vi "teleop_v2.vi"() -> ()   [LabVIEW 2012, in "MainProject.lvrbt"]
uses:
  MainProject.lvrbt
  <vilib>/NXT/Hardware/Plugins/Tetrix DC Motor/TetrixDCMotorAddress.ctl
  <vilib>/NXT/Dual Mode Library/Advanced/NXTFlag_Get_String.vi
  <vilib>/FTC/FTC Read Controller Packet.vi
  <vilib>/FTC/FTC Read Button States.vi
  <vilib>/NXT/NXTIO Xnodes/NXTIONodeSubVIs/TETRIX IO Move DC Motors.vi
  <vilib>/NXT/NXTIO Xnodes/NXTIONodeSubVIs/TETRIX IO Stop DC Motors.vi
  <vilib>/FTC/FTC Calculate Drive Power - Tank.vi
  <vilib>/NXT/Dual Mode Library/Advanced/NXTFlag_Assign_String.vi
  <vilib>/NXT/NXTIO Xnodes/NXTIONodeSubVIs/TETRIX IO Check Battery.vi
  <vilib>/NXT/NXTIO Xnodes/AddressXNode/NXTIOAddress.xnode
  <vilib>/NXT/Subs/LVHSConnector.ctl
  <vilib>/NXT/NXTIO Xnodes/NXTIOXNode/NXTIO.xnode
  <vilib>/NXT/LegoClasses/BrickReference/BrickReference.lvclass
panel:
  in  "Drive Power":i8=75 min=-100 max=100
  # "This VI was generated based on your configuration in the Remote Control Editor. You may modify the code as needed for your robot. To test this program for an FTC match, return to the Remote Control Editor, select the \"Run Program\" tab, and choose \"Teleop\"."
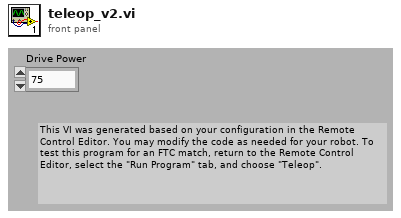
[diagram p1: front panel]
types:
  T1 = typedef "TetrixDCMotorAddress.ctl" = i16
  T2 = cluster{"TetrixDCMotor":T1, "TetrixDCMotor 2":T1}
  T3 = typedef "LVHSConnector.ctl" = refnum<class "BrickReference.lvclass">
  T4 = typedef "FTC ControllerState.ctl" = cluster{"Left X":i8, "Left Y":i8, "Right X":i8, "Right Y":i8, "Button Encoding 9-12":u8, "Button Encoding 1-8":u8, "POV":T5}
  T5 = typedef "FTC POVState.ctl" = i8
  T6 = typedef "FTC ButtonEventType.ctl" = enum16{"Pressed", "Released"}
  T7 = cluster{"Button ID":enum16{"None", "Button 1", "Button 2", "Button 3", "Button 4", "Button 5", "Button 6", "Button 7", "Button 8", "Button 9", "Button 10", "Button 11", "Button 12", "POV Up", "POV Up Right", "POV Right", "POV Down Right", "POV Down", "POV Down Left", "POV Left", "POV Up Left"}, "Event Type":T6}[]
  T8 = enum16{"None", "Button 1", "Button 2", "Button 3", "Button 4", "Button 5", "Button 6", "Button 7", "Button 8", "Button 9", "Button 10", "Button 11", "Button 12", "POV Up", "POV Up Right", "POV Right", "POV Down Right", "POV Down", "POV Down Left", "POV Left", "POV Up Left"}
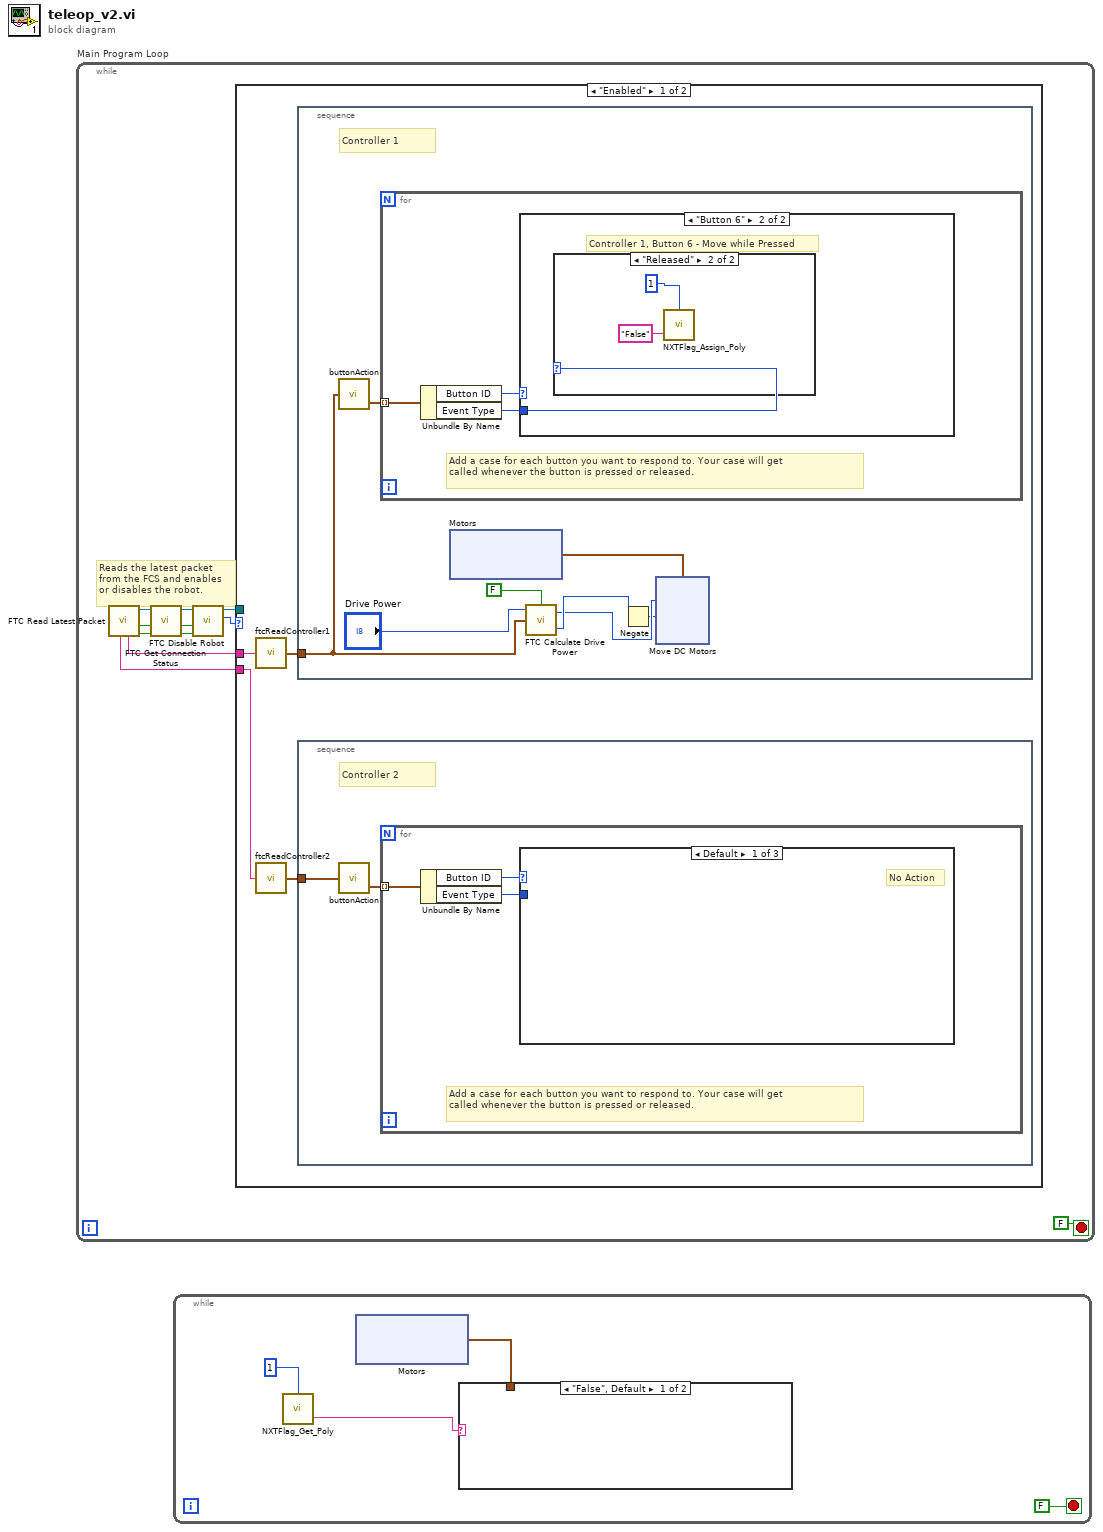
[diagram p0: block diagram]
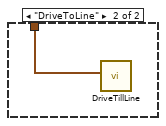
[diagram p2: hidden frame]
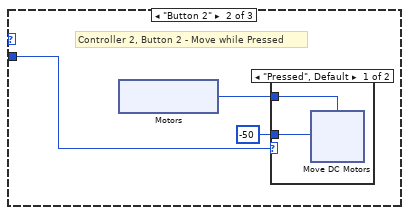
[diagram p3: hidden frame]
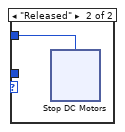
[diagram p4: hidden frame]
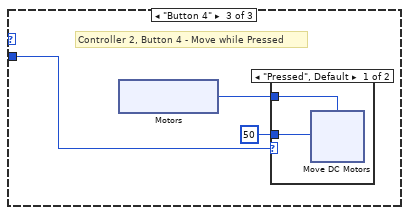
[diagram p5: hidden frame]
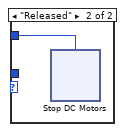
[diagram p6: hidden frame]
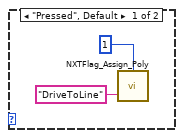
[diagram p8: hidden frame]
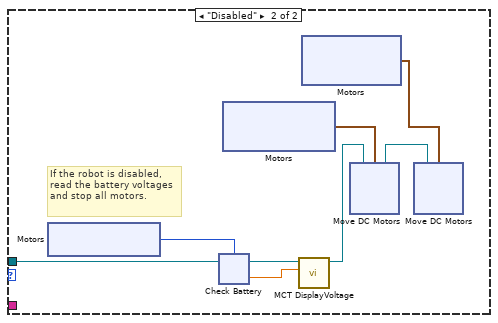
[diagram p9: hidden frame]
diagram:
  n1 = while "Main Program Loop" {
    stop <- FALSE stop-if-true
    # "Reads the latest packet\nfrom the FCS and enables\nor disables the robot."
    n2 = call <vilib>:"FTC Read Latest Packet.vi"() -> ("Packet Received?"=w8:bool, "Stopped?"=w5:bool, "NXT"=w7:T3, "Controller 1"=w10:string, "Controller 2"=w9:string)  [unwired: 6 in, 1 out]
    n3 = call <vilib>:"FTC Get Connection Status.vi"("Packet Received?"=w8, "Stopped?"=w5, "NXT"=w7) -> ("Online?"=w2:bool, "Stopped?"=w3:bool, "NXT"=w4:T3)  [unwired: 5 in]
    n4 = call <vilib>:"FTC Disable Robot.vi"("Online?"=w2, "Stopped?"=w3, "NXT"=w4) -> ("Enabled?"=w6:enum16{"Disabled", "Enabled"}, "NXT"=w1:T3)  [unwired: 3 in]
    n5 = case "disableCase" shown="\"Enabled\"" w6 {
      tunnel: w10 -> [w15 _]
      tunnel: w9 -> [w14 _]
      tunnel: w1 -> [_ w93]
      frame "Enabled" {
        n6 = call "ftcReadController1"("Packet"=w15) -> ("Controller State"=w13:T4)  [unwired: 4 in]
        n7 = call "ftcReadController2"("Packet"=w14) -> ("Controller State"=w12:T4)  [unwired: 4 in]
        n8 = stacked-sequence "controller1Actions" {
          tunnel: w13 -> [w65]
          frame #0 {
            # "Controller 1"
            n9 = call "buttonAction"("Controller State"=w65) -> ("Button Events"=w66:T7)  [unwired: 2 in, 1 out]
            n10 = for "buttonAction" {
              tunnel: w66 -> [w78] mode=indexing
              # "Add a case for each button you want to respond to. Your case will get \ncalled whenever the button is pressed or released."
              n11 = Unbundle By Name(w78) -> ("Button ID"=w80:T8, "Event Type"=w79:T6)
              n12 = case "EventCase1" shown="\"Button 6\"" w80 {
                tunnel: w79 -> [_ w81]
                frame Default {
                  # "No Action"
                }
                frame "Button 6" {
                  # "Controller 1, Button 6 - Move while Pressed"
                  n13 = case shown="\"Released\"" w81 {
                    frame "Pressed", Default {
                      n14 = call-poly <vilib>:"NXTFlag_Assign_Poly.vi"("Flag Value"="DriveToLine", "NXT Flag Number"=i8 1) -> ()  [unwired: 2 in, 1 out]
                    }
                    frame "Released" {
                      n15 = call-poly <vilib>:"NXTFlag_Assign_Poly.vi"("Flag Value"="False", "NXT Flag Number"=i8 1) -> ()  [unwired: 2 in, 1 out]
                    }
                  }
                }
              }
            }
            n16 = xnode "Motors"() -> ("Motor"=w62:cluster{"TetrixDCMotor":T1, "TetrixDCMotor":T1})
            n17 = call-poly <vilib>:"FTC Calculate Drive Power.vi"("Reverse"=FALSE, "Controller State"=w65, "Power Level (50)"="Drive Power") -> ("Right Motor Power"=w61:i8, "Left Motor Power"=w60:i8)  [unwired: 1 in]
            n18 = Negate(x=w61) -> (-x=w59:i8)
            n19 = xnode "Move DC Motors"("Power/Speed 2"=w59, "Power/Speed 1"=w60, "Motors"=w62) -> ()  [unwired: 1 in, 1 out]
          }
        }
        n20 = stacked-sequence "controller2Actions" {
          tunnel: w12 -> [w16]
          frame #0 {
            # "Controller 2"
            n21 = call "buttonAction"("Controller State"=w16) -> ("Button Events"=w17:T7)  [unwired: 2 in, 1 out]
            n22 = for "buttonAction" {
              tunnel: w17 -> [w18] mode=indexing
              # "Add a case for each button you want to respond to. Your case will get \ncalled whenever the button is pressed or released."
              n23 = Unbundle By Name(w18) -> ("Button ID"=w20:T8, "Event Type"=w19:T6)
              n24 = case "EventCase2" shown="Default" w20 {
                tunnel: w19 -> [_ w23 w42]
                frame Default {
                  # "No Action"
                }
                frame "Button 2" {
                  # "Controller 2, Button 2 - Move while Pressed"
                  n25 = xnode "Motors"() -> ("Motor"=w21:T1)
                  n26 = case shown="\"Pressed\", Default" w23 {
                    tunnel: -50 ("Power (75)") -> [w26 _]
                    tunnel: w21 -> [w25 w34]
                    frame "Pressed", Default {
                      n27 = xnode "Move DC Motors"("Power/Speed 1"=w26, "Motors"=w25) -> ()  [unwired: 1 in, 1 out]
                    }
                    frame "Released" {
                      n28 = xnode "Stop DC Motors"("Motors"=w34) -> ()  [unwired: 1 in, 1 out]
                    }
                  }
                }
                frame "Button 4" {
                  # "Controller 2, Button 4 - Move while Pressed"
                  n29 = xnode "Motors"() -> ("Motor"=w40:T1)
                  n30 = case shown="\"Pressed\", Default" w42 {
                    tunnel: 50 ("Power (75)") -> [w45 _]
                    tunnel: w40 -> [w44 w53]
                    frame "Pressed", Default {
                      n31 = xnode "Move DC Motors"("Power/Speed 1"=w45, "Motors"=w44) -> ()  [unwired: 1 in, 1 out]
                    }
                    frame "Released" {
                      n32 = xnode "Stop DC Motors"("Motors"=w53) -> ()  [unwired: 1 in, 1 out]
                    }
                  }
                }
              }
            }
          }
        }
      }
      frame "Disabled" {
        # "If the robot is disabled, read the battery voltages and stop all motors."
        n33 = xnode ("Motors")() -> ("Motor"=w92:T1)
        n34 = xnode ("Check Battery")("Motors"=w92, "NXT"=w93) -> ("Voltage 1"=w91:sgl, "NXT"=w90:T3)
        n35 = xnode "Motors"() -> ("Motor"=w89:cluster{"TetrixDCMotor":T1, "TetrixDCMotor":T1})
        n36 = call <vilib>:"MCT DisplayVoltage.vi"("Motor Voltage"=w91, "NXT"=w90) -> ("NXT"=w88:T3)  [unwired: 9 in]
        n37 = xnode "Motors"() -> ("Motor"=w87:cluster{"TetrixDCMotor":T1, "TetrixDCMotor":T1})
        n38 = xnode "Move DC Motors"("Motors"=w89, "NXT"=w88) -> ("NXT"=w86:T3)
        n39 = xnode "Move DC Motors"("Motors"=w87, "NXT"=w86) -> ()  [unwired: 1 out]
      }
    }
  }
  n40 = while {
    stop <- FALSE stop-if-true
    n41 = call-poly <vilib>:"NXTFlag_Get_Poly.vi"("NXT Flag Number"=1) -> ("Flag Value"=w117:string)  [unwired: 2 in, 1 out]
    n42 = xnode "Motors"() -> ("Motor"=w116:cluster{"TetrixDCMotor":T1, "TetrixDCMotor":T1})
    n43 = case shown="\"False\", Default" w117 {
      tunnel: w116 -> [_ w120]
      frame "False", Default {
      }
      frame "DriveToLine" {
        n44 = call "DriveTillLine.vi"("Motor"=w120) -> ()  [unwired: 10 in, 1 out]
      }
    }
  }
